vi "shm_open.vi"(7 "flags":T1, 8 "error in (no error)":errorcluster, 9 "access mode (read/write)":enum16{"read only", "read and write"}(ring)=enum."read and write", 10 "permissions (0777)":T2=511 format="%04o", 11 "shared memory name":string) -> (0 "error out":errorcluster, 3 "file descriptor":i32)   [LabVIEW 2013, in "Shared Memory.lvlib" / "Shared Memory.lvclass"]
doc: "Wrapper VI for Linux function shm_open()."
uses:
  Shared Memory.lvclass
  Controls/C Types/mode_t.ctl
  Controls/fcntl-linux file modes.ctl
  Controls/functions.ctl
  <vilib>/NI/NI Linux RT Errno/Linux Errno.lvlib
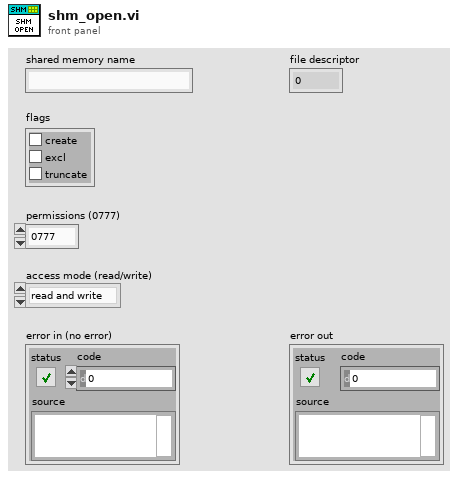
[diagram p1: front panel]
types:
  T1 = cluster{"create":bool, "excl":bool, "truncate":bool}
  T2 = typedef "Shared Memory.lvlib/Shared Memory.lvclass/mode_t.ctl" = u32
  T3 = typedef "Shared Memory.lvlib/Shared Memory.lvclass/functions.ctl" = enum16{"unspecified", "shm_open", "ftruncate", "mmap", "munmap", "close", "shm_unlink", "fstat"}
  T4 = typedef "Shared Memory.lvlib/Shared Memory.lvclass/fcntl-linux file modes.ctl" = u16
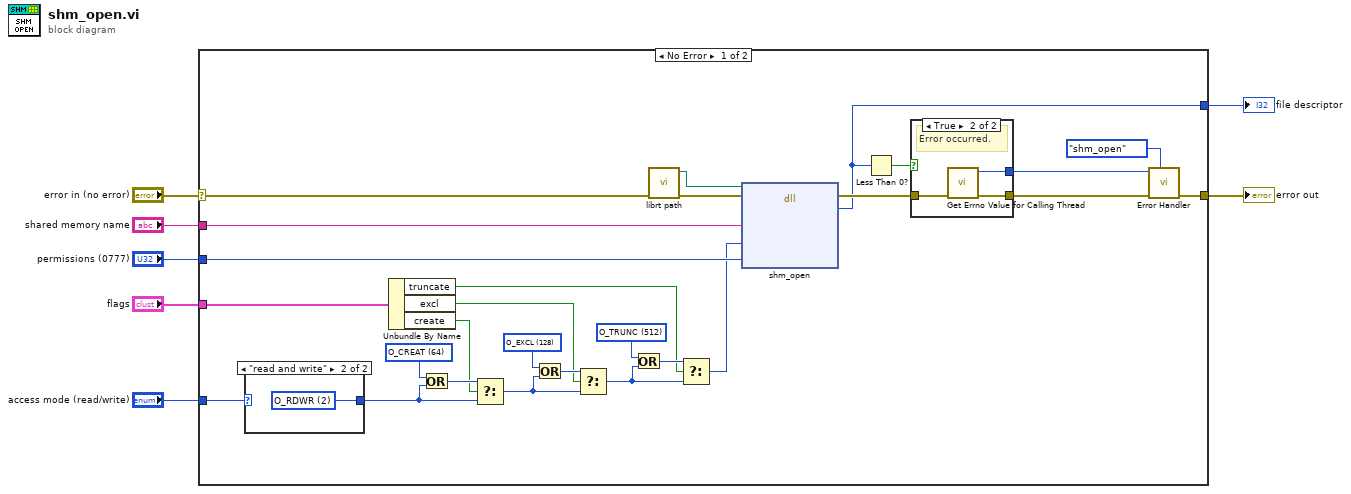
[diagram p0: block diagram]
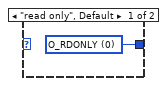
[diagram p2: hidden frame]
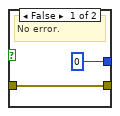
[diagram p3: hidden frame]
diagram:
  n1 = case shown="No Error" "error in (no error)" {
    selector: "error in (no error)" -> [w29 w42]
    tunnel: "shared memory name" -> [w34 _]
    tunnel: "permissions (0777)" -> [w33 _]
    tunnel: [w30 w42] -> w5
    tunnel: [w8 _] -> w4
    tunnel: "flags" -> [w27 _]
    tunnel: "access mode (read/write)" -> [w26 _]
    frame No Error {
      w14 = T4 512 items=["O_RDONLY"=0, "O_WRONLY"=1, "O_RDWR"=2, "O_CREAT"=64, "O_EXCL"=128, "O_TRUNC"=512] ("fcntl")
      w19 = T4 128 items=["O_RDONLY"=0, "O_WRONLY"=1, "O_RDWR"=2, "O_CREAT"=64, "O_EXCL"=128, "O_TRUNC"=512] ("fcntl")
      w22 = T4 64 items=["O_RDONLY"=0, "O_WRONLY"=1, "O_RDWR"=2, "O_CREAT"=64, "O_EXCL"=128, "O_TRUNC"=512] ("fcntl")
      n2 = case shown="\"read and write\"" w26 {
        tunnel: [w35 w36] -> w23
        frame "read only", Default {
          w35 = T4 0 items=["O_RDONLY"=0, "O_WRONLY"=1, "O_RDWR"=2, "O_CREAT"=64, "O_EXCL"=128, "O_TRUNC"=512] ("fcntl")
        }
        frame "read and write" {
          w36 = T4 2 items=["O_RDONLY"=0, "O_WRONLY"=1, "O_RDWR"=2, "O_CREAT"=64, "O_EXCL"=128, "O_TRUNC"=512] ("fcntl")
        }
      }
      n3 = Unbundle By Name(w27) -> ("truncate"=w12:bool, "excl"=w16:bool, "create"=w20:bool)
      n4 = Or(x=w22, y=w23) -> (x .or. y?=w21:T4)
      n5 = Select(t=w21, s=w20, f=w23) -> (s? t:f=w17:T4)
      n6 = Or(x=w19, y=w17) -> (x .or. y?=w18:T4)
      n7 = Select(t=w18, s=w16, f=w17) -> (s? t:f=w13:T4)
      n8 = Or(x=w14, y=w13) -> (x .or. y?=w15:T4)
      n9 = call "librt path.vi"("error in (no error)"=w29) -> ("error out"=w10:errorcluster, "path to librt"=w9:path)  [unwired: 9 in]
      n10 = Select(t=w15, s=w12, f=w13) -> (s? t:f=w11:T4)
      n11 = dll-call lib="?" fn="shm_open"(path in=w9, error in=w10, "name"=w34, "flags"=w11, "mode"=w33) -> (error out=w25:errorcluster, "fd"=w8:i32)  [unwired: 4 in, 1 out]
      n12 = Less Than 0?(x=w8) -> (x < 0?=w24:bool)
      n13 = case shown="True" w24 {
        tunnel: w25 -> [w38 w41]
        tunnel: [w38 w40] -> w31
        tunnel: [0 ("errno") w39] -> w28
        frame False {
          # "No error."
        }
        frame True {
          # "Error occurred."
          n14 = call <vilib>:"Get Errno Value for Calling Thread.vi"("error in (no error)"=w41) -> ("error out"=w40:errorcluster, "errno"=w39:i32)  [unwired: 9 in]
        }
      }
      n15 = call "Error Handler.vi"("function"=functions."shm_open", "error in (no error)"=w31, "errno"=w28) -> ("error out"=w30:errorcluster)  [unwired: 8 in]
    }
    frame Error {
    }
  }
  "error out" <- w5
  "file descriptor" <- w4
